vi "Unix Epoch to LV Timestamp.vi"(10 "Unix Timestamp":u64) -> (2 "LV Timestamp (UTC)":timestamp)   [LabVIEW 2020, in "hse-misc.lvlib"]
doc: "Convert a Unix Epoch Timestamp (C time_t) to a LabView Timestamp (UTC Timezone).\n\n____\nHAMPEL SOFTWARE ENGINEERING v3.8.0 (2023-12-18 14:41)"
uses:
  hse-misc.lvlib
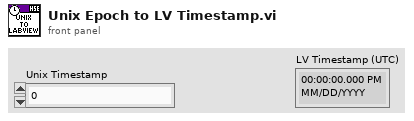
[diagram p1: front panel]
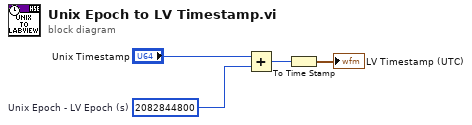
[diagram p0: block diagram]
diagram:
  w4 = u64 2082844800  # Unix Epoch - LV Epoch (s)
  n1 = Add(x="Unix Timestamp", y=w4) -> (x+y=w3:u64)
  n2 = To Time Stamp(1:w3) -> (0:→"LV Timestamp (UTC)":timestamp)
